vi "updateRf.vi"(8 "error in (no error)":errorcluster, 11 "StaticOutputEditor in":refnum<class "StaticOutputEditor.lvclass">) -> (0 "error out":errorcluster, 3 "StaticOutputEditor out":refnum<class "StaticOutputEditor.lvclass">)   [LabVIEW 2011, in "Views.lvlib" / "ScriptEditor.lvlib" / "StaticOutputEditor.lvclass"]
uses:
  StaticOutputEditor.lvclass
  StaticOutputEditor.lvclass/StaticOutputEditor.ctl
  Hal/HWController/HWControllerEvents/HWControllerEvents.lvclass
  Tools/DatabaseHelpers/Database Objects/ChannelArray/ChannelArray.lvclass
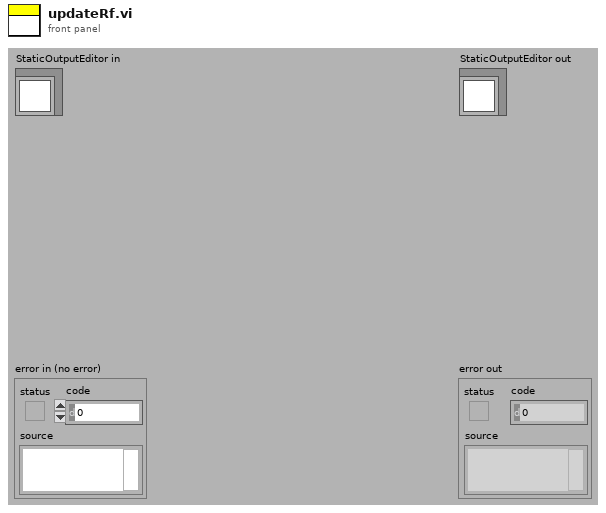
[diagram p1: front panel]
types:
  T1 = enum16{"Sine", "Square", "Triangle", "Arbitrary"}
  T2 = enum16{"start", "stop", "statusInquiry", "configure", "resetError", "resourcesInquiry", "reserveResources", "initialise", "resetAllChannels", "staticUpdate", "close", "HWStatus", "error", "resourcesAvailable", "resourcesReserved", "compilerError", "compiledScript", "compilingScript", "runScript", "configureCompiledScript", "restartCompiler", "staticRfChannelUpdate"}
  T3 = cluster{"channelName":string, "value":string, "freq":string, "phase":string}[]
  T4 = cluster{"channelName":string, "value":string, "freq":string, "phase":string}
  T5 = cluster{"incomingEventTypes":cluster{"start":cluster{"Boolean":bool}, "stop":cluster{"Boolean":bool}, "statusInquiry":cluster{"Boolean":bool}, "configure":cluster{"DPScriptPath":path, "TimeStamp":string, "HWLoop?":bool}, "resetError":cluster{"Boolean":bool}, "resourcesInquiry":cluster{"Boolean":bool}, "reserveResources":cluster{"HWList":string[]}, "initialise":cluster{"HWList":string[]}, "close":cluster{"Boolean":bool}, "resetAllChannels":cluster{"Boolean":bool}, "staticChannelUpdate":cluster{"channel_address":string, "calibratedValue":dbl}, "runScript":cluster{"DPScriptPath":path, "TimeStamp":string, "HWLoop?":bool}, "compilingScript":cluster{"Path":path}, "compiledScript":cluster{"Path":path, "timeCompileAt":string}, "compilerError":cluster{"Path":path}, "configureCompiledScript":cluster{"DPScriptPath":path, "TimeStamp":string, "HWLoop?":bool, "CompiledScript":cluster{"ScriptListCompiler.lvclass":refnum<class "ScriptListCompiler.lvclass">, "aoChannels":refnum<class "AnalogOutput.lvclass">[], "doChannels":refnum<class "DigitalOutput.lvclass">[], "rfChannels":refnum<class "DDSOutput.lvclass">[]}}, "restartCompiler":cluster{"restart":bool}, "staticRfChannelUpdate":cluster{"channel_address":string, "Output":cluster{"Frequency(MHz)":dbl, "Amplitude":dbl, "Phase":dbl, "OutputForm":enum16{"Sine", "Square", "Triangle", "Arbitrary"}}}, "cameraUpdate":cluster{"Camera":string, "Type":string, "settings":path}}, "outgoingEventTypes":cluster{"HWStatus":cluster{"status":enum16{"Ready", "Compiling", "Configured", "Running", "Stopping", "Unresolved Error"}}, "error":cluster{"error out":errorcluster}, "resourcesAvailable":cluster{"availableHWList":string[], "reservedHWList":string[]}, "resourcesReserved":cluster{"reservedHWList":string[]}}}
  T6 = cluster{"channel_address":string, "Output":cluster{"Frequency(MHz)":dbl, "Amplitude":dbl, "Phase":dbl, "OutputForm":enum16{"Sine", "Square", "Triangle", "Arbitrary"}}}
  T7 = cluster{"eventId":enum16{"start", "stop", "statusInquiry", "configure", "resetError", "resourcesInquiry", "reserveResources", "initialise", "resetAllChannels", "staticUpdate", "close", "HWStatus", "error", "resourcesAvailable", "resourcesReserved", "compilerError", "compiledScript", "compilingScript", "runScript", "configureCompiledScript", "restartCompiler", "staticRfChannelUpdate"}, "staticRfChannelUpdate":cluster{"channel_address":string, "Output":cluster{"Frequency(MHz)":dbl, "Amplitude":dbl, "Phase":dbl, "OutputForm":enum16{"Sine", "Square", "Triangle", "Arbitrary"}}}}
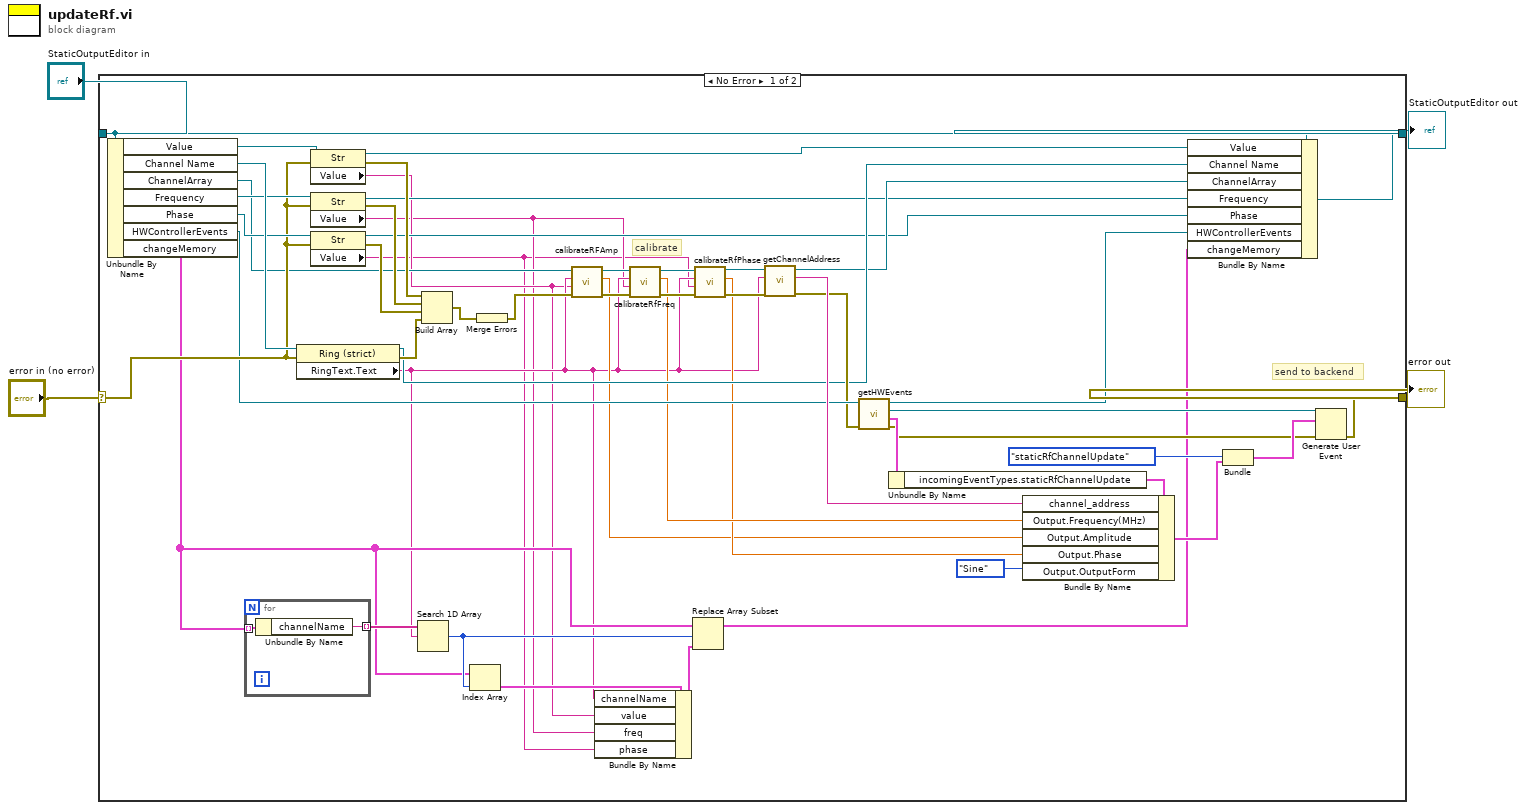
[diagram p0: block diagram]
diagram:
  n1 = case shown="No Error" "error in (no error)" {
    selector: "error in (no error)" -> [w43 w59]
    tunnel: [w55 w59] -> w3
    tunnel: [w15 w58] -> w1
    tunnel: "StaticOutputEditor in" -> [w24 w58]
    frame No Error {
      # "calibrate"
      # "send to backend"
      n2 = Unbundle By Name(w24) -> ("Value"=w53:refnum<vi>, "Channel Name"=w54:refnum<vi>, "ChannelArray"=w32:refnum<class "ChannelArray.lvclass">, "Frequency"=w45:refnum<vi>, "Phase"=w44:refnum<vi>, "HWControllerEvents"=w29:refnum<class "HWControllerEvents.lvclass">, "changeMemory"=w12:T3)
      n3 = for {
        tunnel: w12 -> [w56] mode=indexing
        tunnel: [w57] -> w14 mode=indexing
        n4 = Unbundle By Name(w56) -> ("channelName"=w57:string)
      }
      n5 = property class="Ring (strict)"(reference=w54, error in=w43) -> (reference out=w25:refnum<vi>, error out=w35:errorcluster, "RingText.Text"=w10:string)
      n6 = property class="Str"(reference=w53, error in=w43) -> (reference out=w48:refnum<vi>, error out=w38:errorcluster, "Value"=w9:string)
      n7 = property class="Str"(reference=w45, error in=w43) -> (reference out=w21:refnum<vi>, error out=w37:errorcluster, "Value"=w8:string)
      n8 = property class="Str"(reference=w44, error in=w43) -> (reference out=w20:refnum<vi>, error out=w36:errorcluster, "Value"=w7:string)
      n9 = Search 1D Array(1D array=w14, element=w10) -> (index of element=w13:i32)  [unwired: 1 in]
      n10 = Build Array(w38, w37, w36, w35) -> (w33:errorcluster[])
      n11 = Index Array(array=w12, index=w13) -> (element=w11:T4)
      n12 = Merge Errors(w33) -> (w34:errorcluster)
      n13 = call "calibrateRFAmp.vi"("error in (no error)"=w34, "amplitude"=w9, "channel_name"=w10, "ChannelArray in"=w32) -> ("error out"=w40:errorcluster, "amplitude"=w16:dbl, "ChannelArray out"=w42:refnum<class "ChannelArray.lvclass">)  [unwired: 5 in]
      n14 = Bundle By Name(cluster=w11, "channelName"=w10, "value"=w9, "freq"=w8, "phase"=w7) -> (w6:T4)
      n15 = call "calibrateRfFreq.vi"("error in (no error)"=w40, "amplitude"=w8, "channel_name"=w10, "ChannelArray in"=w42) -> ("error out"=w39:errorcluster, "frequency"=w18:dbl, "ChannelArray out"=w41:refnum<class "ChannelArray.lvclass">)  [unwired: 5 in]
      n16 = Replace Array Subset(array=w12, new element=w6, index=w13) -> (w5:T3)
      n17 = call "calibrateRfPhase.vi"("error in (no error)"=w39, "amplitude"=w7, "channel_name"=w10, "ChannelArray in"=w41) -> ("error out"=w30:errorcluster, "phase"=w17:dbl, "ChannelArray out"=w31:refnum<class "ChannelArray.lvclass">)  [unwired: 5 in]
      n18 = call "getChannelAddress.vi"("error in (no error)"=w30, "channel_name"=w10, "ChannelArray in"=w31) -> ("error out"=w28:errorcluster, "channel_address"=w52:string, "ChannelArray out"=w23:refnum<class "ChannelArray.lvclass">)  [unwired: 6 in]
      n19 = call-dynamic "getHWEvents.vi"("error in (no error)"=w28, "HWControllerEvents in"=w29) -> ("error out"=w19:errorcluster, "eventDataTypes"=w27:T5, "HWCEvent"=w49:refnum<user-event>, "HWControllerEvents out"=w22:refnum<class "HWControllerEvents.lvclass">)  [unwired: 6 in]
      n20 = Unbundle By Name(w27) -> ("incomingEventTypes.staticRfChannelUpdate"=w26:T6)
      n21 = Bundle By Name(cluster=w26, "channel_address"=w52, "Output.Frequency(MHz)"=w18, "Output.Amplitude"=w16, "Output.Phase"=w17, "Output.OutputForm"=T1."Sine") -> (w51:T6)
      n22 = Bundle By Name(cluster=w24, "Value"=w48, "Channel Name"=w25, "ChannelArray"=w23, "Frequency"=w21, "Phase"=w20, "HWControllerEvents"=w22, "changeMemory"=w5) -> (w15:refnum<class "StaticOutputEditor.lvclass">)
      n23 = Bundle("eventId"=T2."staticRfChannelUpdate", "staticRfChannelUpdate"=w51) -> (w50:T7)  [unwired: 1 in]
      n24 = Generate User Event(user event=w49, event data cluster=w50, error in=w19) -> (error out=w55:errorcluster)  [unwired: 1 out]
    }
    frame Error {
    }
  }
  "error out" <- w3
  "StaticOutputEditor out" <- w1
